vi "dfd_Validate NStage MRate for Plot.vi"(8 "error in (no error)":errorcluster, 11 "multirate filters in":T1[](array[typedef]) {"mMRate_SumWl" min=1 max=32 step=1; "mMRate_InputIwl" min=1 max=32 step=1; "mMRate_GainWl" min=1 max=32 step=1; "mMRate_OutputWl" min=1 max=32 step=1; "mMRate_InputWl" min=1 max=32 step=1; "mMRate_CoefWl" min=1 max=32 step=1; "mMRate_Mode" items=["Default"=-1, "No Rate Change"=0, "Interpolation"=1, "Decimation"=2, "Interpolated"=3, "Rational"=4]}) -> (0 "error out":errorcluster, 3 "multirate filters out":T1[](array[typedef]) {"mMRate_SumWl" min=1 max=32 step=1; "mMRate_InputIwl" min=1 max=32 step=1; "mMRate_GainWl" min=1 max=32 step=1; "mMRate_OutputWl" min=1 max=32 step=1; "mMRate_InputWl" min=1 max=32 step=1; "mMRate_CoefWl" min=1 max=32 step=1; "mMRate_Mode" items=["Default"=-1, "No Rate Change"=0, "Interpolation"=1, "Decimation"=2, "Interpolated"=3, "Rational"=4]})   [LabVIEW 2017, in "NI_DigFilterLicensed.lvlib"]
uses:
  <vilib>/addons/Digital Filter Design/NI_DigFilterLicensed.lvlib
  <vilib>/addons/Digital Filter Design/_Objects.llb/DFD Multirate Filter Obj.ctl
  <vilib>/addons/Digital Filter Design/_Objects.llb/DFD Multirate Mode.ctl
  <vilib>/addons/Digital Filter Design/_Objects.llb/DFD Coef Norm Type.ctl
  <vilib>/addons/Digital Filter Design/_Objects.llb/DFD Round-off Mode.ctl
  <vilib>/addons/Digital Filter Design/_Objects.llb/DFD FXP MRate Multiply Mode.ctl
  <vilib>/addons/Digital Filter Design/_Misc.llb/dfd_Error Handlers (Single).vi
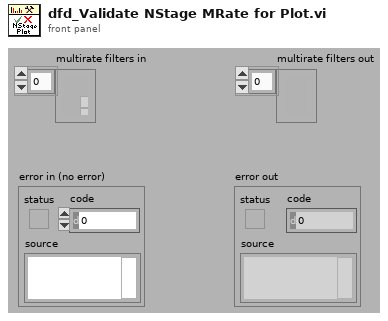
[diagram p1: front panel]
types:
  T1 = typedef "NI_DigFilterLicensed.lvlib/DFD Multirate Filter Obj.ctl" = cluster{"mMRate_Structure":enum16{"CIC", "FIR", "IIR", "Lattice"}, "mMRate_Mode":T2, "mMRate_Factor":i32, "mMRate_FIRParams":cluster{"mMRate_FIR_H":dbl[], "mMRate_FIR_IsNyquist?":bool, "mMRate_FIR_IsSymmetric?":bool}, "mMRate_CICParams":cluster{"mMRate_CIC_#Stage":i32, "mMRate_CIC_Lag":i32, "mMRate_CIC_Type":enum16{"Lowpass", "Highpass"}}, "mMRate_Order":i32, "mMRate_Version":string, "mMRate_Comments":string, "mMRate_RationalFactor":cluster{"mMRate_L":i32, "mMRate_M":i32}, "mMRate_Fs":dbl, "mMRate_Quantized?":bool, "mMRate_QFilterGain":dbl, "mMRate_CoefWl":i16, "mMRate_Scaling":cluster{"mMRate_ScaleByPowerOf2?":bool, "mMRate_ScaleType":T3}, "mMRate_InputWl":i16, "mMRate_OutputWl":i16, "mMRate_OutputMode":T4, "mMRate_MultMode":T5, "mMRate_BitPruning":bool, "mMRate_GainWl":i16, "mMRate_OutputFwl":i16, "mMRate_SumIwl":i16, "mMRate_InputIwl ":i16, "mMRate_SumWl":i16, "mMRate_CoefIwl":i16}
  T2 = typedef "NI_DigFilterLicensed.lvlib/DFD Multirate Mode.ctl" = i16
  T3 = typedef "NI_DigFilterLicensed.lvlib/DFD Coef Norm Type.ctl" = enum16{"No Norm", "Time Domain 1-Norm", "Time Domain 2-Norm", "Time Domain Inf-Norm"}
  T4 = typedef "NI_DigFilterLicensed.lvlib/DFD Round-off Mode.ctl" = enum16{"Nearest", "Truncation"}
  T5 = typedef "NI_DigFilterLicensed.lvlib/DFD FXP MRate Multiply Mode.ctl" = enum16{"Truncated", "Full"}
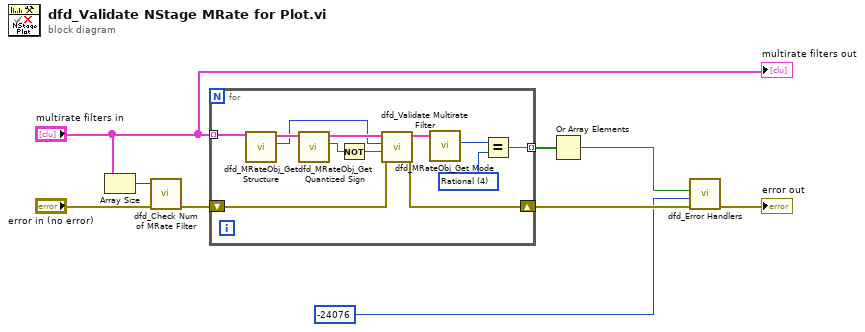
[diagram p0: block diagram]
diagram:
  n1 = Array Size(array="multirate filters in") -> (size(s)=w6:i32)
  n2 = call <vilib>:"dfd_Check Num of MRate Filter.vi"("error in (no error)"="error in (no error)", "#MRate in"=w6) -> ("error out"=w3:errorcluster)  [unwired: 9 out]
  n3 = for {
    tunnel: "multirate filters in" -> [w13] mode=indexing
    shift-right: [w12] -> w8
    shift-left: w3 -> [w10]
    tunnel: [w19] -> w9 mode=indexing
    w20 = T2 4 items=["Default"=-1, "No Rate Change"=0, "Interpolation"=1, "Decimation"=2, "Interpolated"=3, "Rational"=4] ("y")
    n4 = call <vilib>:"dfd_MRateObj_Get Structure.vi"("multirate filter in"=w13) -> ("structure"=w14:enum16{"CIC", "FIR", "IIR", "Lattice"}, "dup multirate filter"=w15:T1)  [unwired: 9 out]
    n5 = call <vilib>:"dfd_MRateObj_Get Quantized Sign.vi"("multirate filter in"=w15) -> ("is Quantized?"=w17:bool, "dup multirate filter"=w18:T1)  [unwired: 9 out]
    n6 = Not(x=w17) -> (.not. x?=w16:bool)
    n7 = call <vilib>:"dfd_Validate Multirate Filter.vi"("error in (no error)"=w10, "skip FXP? (T)"=w16, "preferred structure"=w14, "multirate filter in"=w18) -> ("error out"=w12:errorcluster, "multirate filter out"=w11:T1)  [unwired: 6 out]
    n8 = call <vilib>:"dfd_MRateObj_Get Mode.vi"("multirate filter in"=w11) -> ("mode"=w21:T2)  [unwired: 10 out]
    n9 = Equal?(x=w21, y=w20) -> (x = y?=w19:bool)
  }
  n10 = Or Array Elements(Boolean array=w9) -> (logical OR=w2:bool)
  n11 = call-poly <vilib>:"dfd_Error Handlers.vi"("error in (no error)"=w8, "error code"=-24076 ("ERR_CANT_PLOT_RATIONAL_NSTAGE"), "condition failed?"=w2) -> ("error out"=→"error out":errorcluster)  [unwired: 8 out]
  "multirate filters out" <- "multirate filters in"
